vi "01 Reading a voltage.vi"() -> ()   [LabVIEW 2019]
uses:
  <vilib>/httpClient/LabVIEWHTTPClient.lvlib
panel:
  out "Temperature (C)":dbl(knob) scale=0.0..40.0
  # "Hit the Run arrow and see the Gauge change to the temperature reading\n\nHit Continuous Run and watch the Gauge change as the temperature changes\n\nUse http://iot.seeed.cc to set up your WIO"
  # "Hit Cmd E to see the diagram (code)"
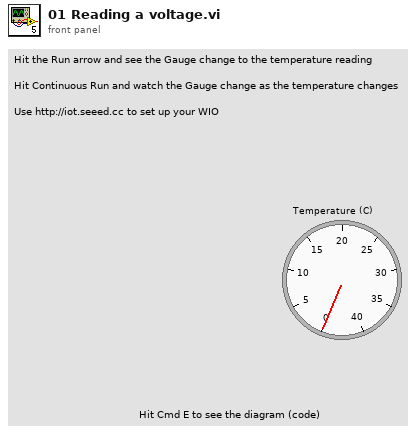
[diagram p1: front panel]
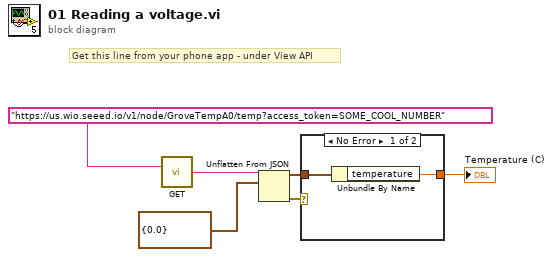
[diagram p0: block diagram]
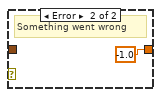
[diagram p2: hidden frame]
diagram:
  # "Get this line from your phone app - under View API"
  n1 = call <vilib>:"GET.vi"("url"="https://us.wio.seeed.io/v1/node/GroveTempA0/temp?access_token=SOME_COOL_NUMBER") -> ("body"=w3:string)  [unwired: 11 in, 3 out]
  n2 = Unflatten From JSON(JSON string=w3, type and defaults=cluster{"temperature":dbl} {"temperature"=0.0}) -> (value=w5:cluster{"temperature":dbl}, error out=w4:errorcluster)  [unwired: 5 in]
  n3 = case shown="No Error" w4 {
    tunnel: w5 -> [w8 _]
    tunnel: [w7 -1.0 ("temperature")] -> w1
    frame No Error {
      n4 = Unbundle By Name(w8) -> ("temperature"=w7:dbl)
    }
    frame Error {
      # "Something went wrong"
    }
  }
  "Temperature (C)" <- w1
